vi "To String.vi"(8 "error in (no error)":errorcluster, 10 "Parameters":variant, 11 "AbstractData in":refnum<class "AbstractData.lvclass">) -> (0 "error out":errorcluster, 2 "String":string, 3 "AbstractData out":refnum<class "AbstractData.lvclass">)   [LabVIEW 2014, in "AbstractData.lvclass"]
uses:
  AbstractData.lvclass
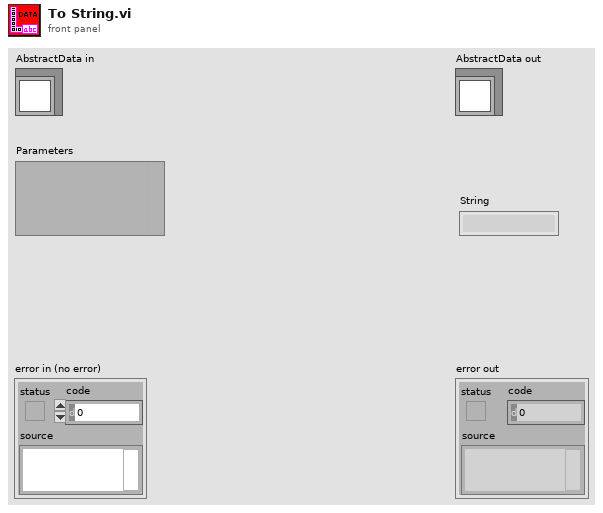
[diagram p1: front panel]
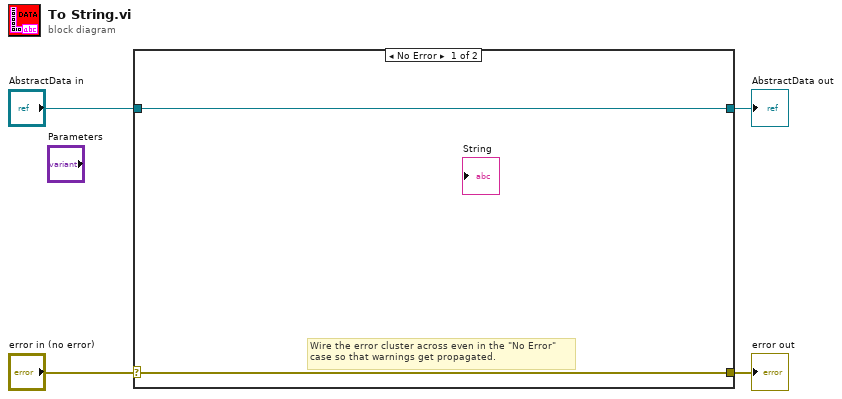
[diagram p0: block diagram]
diagram:
  n1 = case shown="No Error" "error in (no error)" {
    selector: "error in (no error)" -> [w6 w8]
    tunnel: [w6 w8] -> w3
    tunnel: [w5 w7] -> w1
    tunnel: "AbstractData in" -> [w5 w7]
    frame No Error {
      # "Wire the error cluster across even in the \"No Error\"\ncase so that warnings get propagated."
    }
    frame Error {
    }
  }
  "error out" <- w3
  "AbstractData out" <- w1
